vi "Clear Unit of Work.vi"(8 "error in (no error)":errorcluster, 11 "Entity Manager in":refnum<class "Entity Manager.lvclass">) -> (0 "error out":errorcluster, 3 "Entity Manager out":refnum<class "Entity Manager.lvclass">)   [LabVIEW 2020, in "Conditum.lvlib" / "Entity Manager.lvclass"]
doc: "Empties the Unit of Work cache so that entity lookups are forced to query the database the next time a specific entity is looked up by ID."
uses:
  Entity Manager.lvclass
  Entity Manager.lvclass/Entity Manager.ctl
  Unit Of Work Session/Unit Of Work Session.lvclass
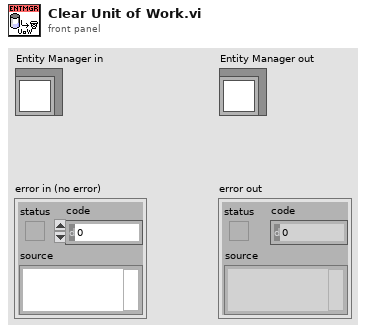
[diagram p1: front panel]
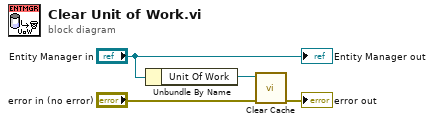
[diagram p0: block diagram]
diagram:
  n1 = Unbundle By Name("Entity Manager in") -> ("Unit Of Work"=w3:refnum<class "Unit Of Work Session.lvclass">)
  n2 = call "Clear Cache.vi"("error in (no error)"="error in (no error)", "Unit Of Work in"=w3) -> ("error out"=→"error out":errorcluster)  [unwired: 9 in]
  "Entity Manager out" <- "Entity Manager in"
